vi "Initialize.vi"(7 "Serial Configuration":T1={"Baud Rate"=9600, "Parity"=0, "Data Bits"=8, "Stop Bits"=10, "Flow Control"=0, "Remote Channel"="CH 1"} {"Flow Control" items=["None", "XON/XOFF", "RTS/CTS", "XON/XOFF & RTS/CTS", "DTR/DSR", "XON/XOFF & DTR/DSR"]; "Stop Bits" items=["1.0"=10, "1.5"=15, "2.0"=20]; "Data Bits" items=["7"=7, "8"=8]; "Parity" items=["None", "Odd", "Even", "Mark", "Space"]; "Baud Rate" items=["300"=300, "600"=600, "1200"=1200, "2400"=2400, "4800"=4800, "9600"=9600, "19200"=19200]}, 8 "error in (no error)":errorcluster, 10 "ID Query (True)":bool, 11 "VISA resource name":refnum<visa-resource-name>) -> (0 "error out":errorcluster, 2 "Inst Info":string, 3 "VISA resource name out":refnum<visa-resource-name>)   [LabVIEW 2017, in "ScientiFic DC Power Supply.lvlib"]
doc: "Establishes communication with the instrument and optionally performs an instrument identification query and/or an instrument reset. It also places the instrument in a default state needed for other instrument driver operations. Therefore, call this VI before calling other instrument driver VIs for this instrument. Generally, you need to call the <b>Initialize</b> VI only once at the beginning of an application."
uses:
  ScientiFic DC Power Supply.lvlib
  <vilib>/Instr/_visa.llb/VISA Configure Serial Port (Instr).vi
panel:
  # "(c) 2021 <ScientiFic Mes Technik Pvt Ltd>.  ALL RIGHTS RESERVED."
  # "Note: Change control description to remove example text for buses not supported."
  # "Note: Serial settings must match those on the physical instrument.  Review user's manual to determine the correct Flow Control protocol for the instrument.  \"None\" is the least robust option for this setting, and could lead to unreliable data transmission."
  # "Note: If your instrument does not support ID query or Reset, remove the ID Query or Reset control from the front panel and delete the case structure with the ID Query or Reset code from the block diagram."
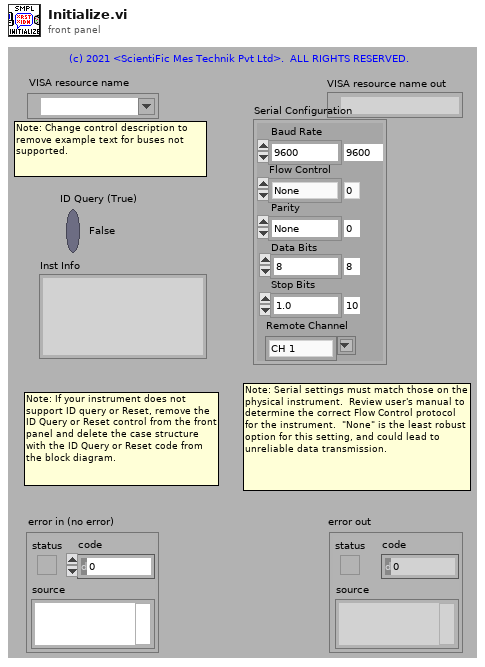
[diagram p1: front panel]
types:
  T1 = cluster{"Baud Rate":u32, "Parity":u16, "Data Bits":u16, "Stop Bits":u16, "Flow Control":u16, "Remote Channel":string}
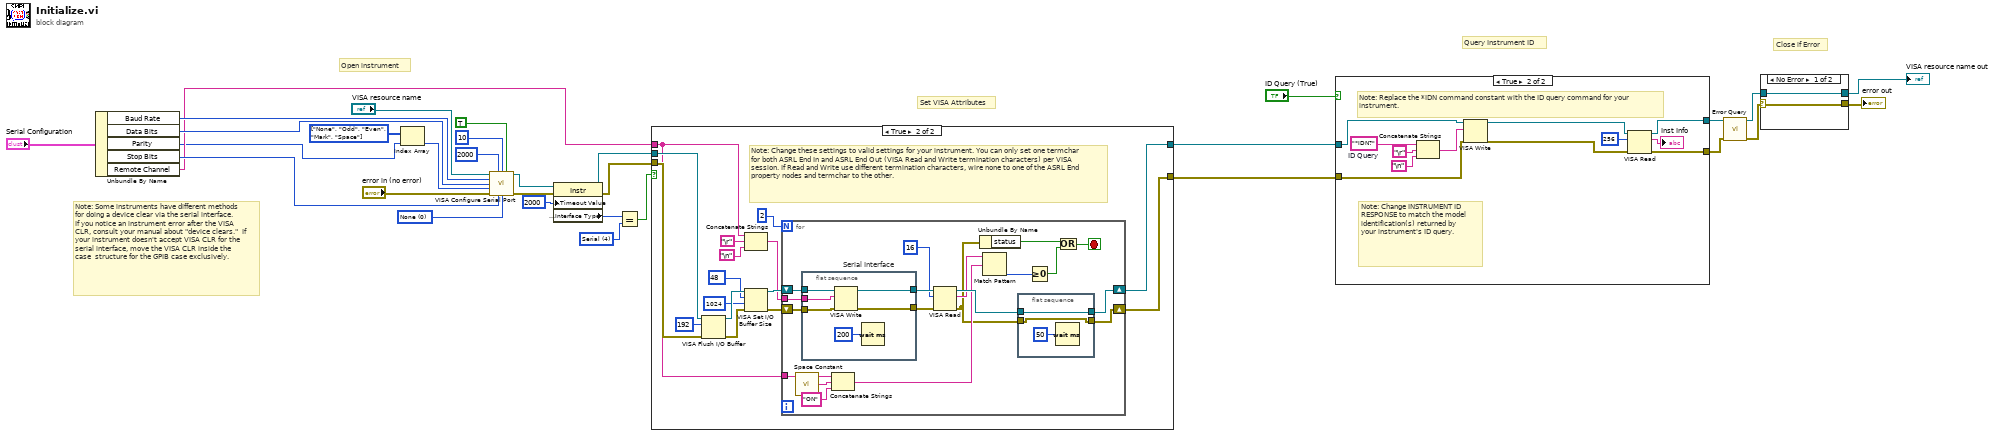
[diagram p0: block diagram]
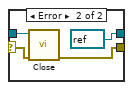
[diagram p2: hidden frame]
diagram:
  w9 = enum16{"None", "Odd", "Even", "Mark", "Space"}[] [enum."None", enum."Odd", enum."Even", enum."Mark", enum."Space"] items=["None", "Odd", "Even", "Mark", "Space"] ("parity (0:none)")
  w11 = u16 0 items=["None", "XON/XOFF", "RTS/CTS", "XON/XOFF & RTS/CTS", "DTR/DSR", "XON/XOFF & DTR/DSR"] ("flow control (0:none)")
  w23 = u16 4 items=["GPIB"=1, "VXI"=2, "GPIB-VXI"=3, "Serial"=4, "PXI"=5, "TCPIP"=6, "USB"=7] ("Interface Information:Interface Type")
  # "Note: Some instruments have different methods for doing a device clear via the serial interface.   If you notice an instrument error after the VISA CLR, consult your manual about \"device clears.\"  If your instrument doesn't accept VISA CLR for the serial interface, move the VISA CLR inside the case  structure for the GPIB case exclusively."
  # "Set VISA Attributes"
  # "Close if Error"
  # "Query Instrument ID"
  # "Open instrument"
  n1 = Unbundle By Name("Serial Configuration") -> ("Baud Rate"=w19:u32, "Data Bits"=w18:u16, "Parity"=w8:u16, "Stop Bits"=w17:u16, "Remote Channel"=w10:string)
  n2 = Index Array(array=w9, index=w8) -> (element=w7:enum16{"None", "Odd", "Even", "Mark", "Space"})
  n3 = call-poly "VISA Configure Serial Port"("VISA resource name"="VISA resource name", "timeout (10sec)"=u32 2000, "termination char\n(0xA = '\\n' = LF)"=u8 10 ("termination char\n(0xA = '\\n' = LF)"), "Enable Termination\nChar (T)"=TRUE ("Enable Termination\nChar (T)"), "baud rate (9600)"=w19, "data bits (8)"=w18, "parity (0:none)"=w7, "error in (no error)"="error in (no error)", "stop bits (10: 1 bit)"=w17, "flow control (0:none)"=w11) -> ("VISA resource name out"=w16:refnum<visa-resource-name>, "error out"=w15:errorcluster)  [unwired: 4 in]
  n4 = property class="Instr"(reference=w16, error in=w15, "General Settings:Timeout Value"=u32 2000) -> (reference out=w26:refnum<visa-resource-name>, error out=w25:errorcluster, "Interface Information:Interface Type"=w30:u16)
  n5 = Equal?(x=w30, y=w23) -> (x = y?=w24:bool)
  n6 = case shown="True" w24 {
    tunnel: [w32 w45] -> w28
    tunnel: [w33 w44] -> w27
    tunnel: w26 -> [w32 w49]
    tunnel: w25 -> [w33 w48]
    tunnel: w10 -> [_ w35]
    frame False {
      # "EDIT: Remove interfaces not supported by your instrument."
      # "GPIB, TCP/IP, and USB Interface"
    }
    frame True {
      # "Note: Change these settings to valid settings for your instrument. You can only set one termchar for both ASRL End In and ASRL End Out (VISA Read and Write termination characters) per VISA session. If Read and Write use different termination characters, wire none to one of the ASRL End property nodes and termchar to the other."
      n7 = VISA Flush I/O Buffer(VISA resource name=w49, mask (16)=u16 192, error in (no error)=w48) -> (VISA resource name out=w40:refnum<visa-resource-name>, error out=w39:errorcluster)
      n8 = Concatenate Strings(w35, "\r", "\n") -> (w41:string)
      n9 = VISA Set I/O Buffer Size(VISA resource name=w40, mask (16)=u16 48, size (4096)=u32 1024 ("size (0)"), error in (no error)=w39) -> (VISA resource name out=w46:refnum<visa-resource-name>, error out=w47:errorcluster)
      n10 = for {
        N: 2 -> [_]
        tunnel: w41 -> [w60]
        tunnel: w35 -> [w58]
        shift-right: [w61] -> w44
        shift-left: w47 -> [w68]
        shift-right: [w62] -> w45
        shift-left: w46 -> [w67]
        stop <- w50 stop-if-true
        # "Serial Interface"
        n11 = call <vilib>:"Space Constant.vi"() -> ("String"=w57:string)
        n12 = flat-sequence {
          tunnel: w68 -> [w74]
          tunnel: w67 -> [w73]
          tunnel: [w72] -> w66
          tunnel: [w71] -> w65
          tunnel: w60 -> [w70]
          frame #0 {
            n13 = VISA Write(VISA resource name=w73, write buffer=w70, error in (no error)=w74) -> (VISA resource name out=w71:refnum<visa-resource-name>, error out=w72:errorcluster)  [unwired: 1 out]
            n14 = Wait (ms)(milliseconds to wait=u32 200) -> ()  [unwired: 1 out]
          }
        }
        n15 = Concatenate Strings(w58, w57, "ON" ("string")) -> (w55:string)
        n16 = VISA Read(VISA resource name=w65, byte count=u32 16, error in (no error)=w66) -> (VISA resource name out=w63:refnum<visa-resource-name>, read buffer=w59:string, error out=w53:errorcluster)  [unwired: 1 out]
        n17 = Unbundle By Name(w53) -> ("status"=w52:bool)
        n18 = Match Pattern(string=w59, regular expression=w55) -> (offset past match=w54:i32)  [unwired: 1 in, 3 out]
        n19 = flat-sequence {
          tunnel: w63 -> [w76]
          tunnel: w53 -> [w75]
          tunnel: [w76] -> w62
          tunnel: [w75] -> w61
          frame #0 {
            n20 = Wait (ms)(milliseconds to wait=u32 50) -> ()  [unwired: 1 out]
          }
        }
        n21 = Greater Or Equal To 0?(x=w54) -> (x >= 0?=w51:bool)
        n22 = Or(x=w52, y=w51) -> (x .or. y?=w50:bool)
      }
    }
  }
  n23 = case shown="True" "ID Query (True)" {
    tunnel: [w78 w81] -> w2
    tunnel: [w79 w89] -> w4
    tunnel: w28 -> [w79 w90]
    tunnel: w27 -> [w78 w91]
    frame False {
    }
    frame True {
      w82 = "*IDN?"  # ID Query
      # "Note: Change INSTRUMENT ID RESPONSE to match the model identification(s) returned by your instrument's ID query."
      # "Note: Replace the *IDN command constant with the ID query command for your instrument."
      n24 = Concatenate Strings(w82, "\r", "\n") -> (w83:string)
      n25 = VISA Write(VISA resource name=w90, write buffer=w83, error in (no error)=w91) -> (VISA resource name out=w88:refnum<visa-resource-name>, error out=w87:errorcluster)  [unwired: 1 out]
      n26 = VISA Read(VISA resource name=w88, byte count=u32 256, error in (no error)=w87) -> (VISA resource name out=w89:refnum<visa-resource-name>, read buffer=→"Inst Info":string, error out=w81:errorcluster)  [unwired: 1 out]
    }
  }
  n27 = call "Error Query.vi"("error in (no error)"=w2, "VISA resource name"=w4) -> ("error out"=w1:errorcluster, "VISA resource name out"=w3:refnum<visa-resource-name>)  [unwired: 8 in]
  n28 = case shown="No Error" w1 {
    selector: w1 -> [w93 w96]
    tunnel: [w92 refnum<visa-resource-name> refnum ("VISA resource name out")] -> w6
    tunnel: [w93 w97] -> w5
    tunnel: w3 -> [w92 w94]
    frame No Error {
    }
    frame Error {
      n29 = call "Close.vi"("error in (no error)"=w96, "VISA resource name"=w94) -> ("error out"=w97:errorcluster)  [unwired: 9 in]
    }
  }
  "VISA resource name out" <- w6
  "error out" <- w5
